vi "DIMPowerSupply.GetRanges.vi"(0 "i ref in":refnum<vi>, 5 "error in (no error)":errorcluster) -> (14 "i ref out":refnum<vi>, 15 "ControlRanges":T1={"deviceMin"=0.0, "deviceMax"=0.0, "numberMin"=0, "numberMax"=0, "U16?"=FALSE, "factor"=1.0} {"deviceMax" format="%.2f"; "deviceMin" format="%.2f"}, 16 "MonitorRanges":T1={"deviceMin"=0.0, "deviceMax"=0.0, "numberMin"=0, "numberMax"=0, "U16?"=FALSE, "factor"=1.0} {"deviceMax" format="%.2f"; "deviceMin" format="%.2f"}, 19 "error out":errorcluster)   [LabVIEW 2014, in "DIMPowerSupply.lvlib"]
doc: "Obtains the ranges of\n1)DeviceMin (minimum voltage value of the power supply output)\n2)DeviceMax (maximum voltage value of the power supply output)\n3)NumberMin (minimum u16 value of the DAC/ADC module)\n4)NumberMax(maximum u16 value of the DAC/ADC module)\n5)ModuleMin (minimum voltage value of the DAC/ADC module)\n6)ModuleMax (maximum voltage value of the DAC/ADC module)"
uses:
  DIMPowerSupply.lvlib
  DIMPowerSupply.ranges type.ctl
  CSCore/BaseProcess/BaseProcess.lvlib
panel:
  in  "Monitor":T1={"deviceMin"=0.0, "deviceMax"=0.0, "numberMin"=0, "numberMax"=0, "U16?"=FALSE, "factor"=1.0} {"deviceMax" format="%.2f"; "deviceMin" format="%.2f"}
  in  "Control":T1={"deviceMin"=0.0, "deviceMax"=0.0, "numberMin"=0, "numberMax"=0, "U16?"=FALSE, "factor"=1.0} {"deviceMax" format="%.2f"; "deviceMin" format="%.2f"}
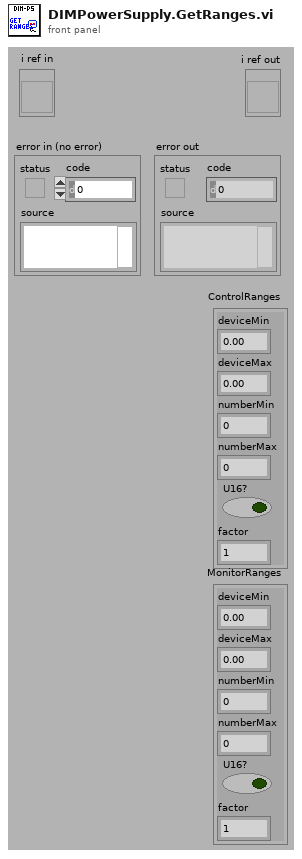
[diagram p1: front panel]
types:
  T1 = typedef "DIMPowerSupply.lvlib/DIMPowerSupply.ranges type.ctl" = cluster{"deviceMin":dbl, "deviceMax":dbl, "numberMin":u16, "numberMax":u16, "U16?":bool, "factor":dbl}
  T2 = typedef "BaseProcess.lvlib/BaseProcess.i attribute.ctl" = cluster{"EventStatus":string, "EventError":i32, "PresetEvtWatchD":i32, "PresetPdcWatchD":i32, "EventTimeout":i32, "PeriodicInterval":i32, "Interface":string[], "Address":string[], "Special":string[], "PeriodicError":i32, "PeriodicStatus":string, "SuperProc":string, "Descriptors":T3[], "CaseRef":refnum<vi>, "PdcRef":refnum<vi>, "Thread Ref":refnum<vi>, "eventErrorID":i32, "eventStatusID":i32, "periodicErrorID":i32, "periodicStatusID":i32, "pdcCtrID":i32}
  T3 = typedef "BaseProcess.lvlib/BaseProcess.descriptor definition.ctl" = cluster{"selector":string, "descriptor":T4}
  T4 = typedef "BaseProcess.lvlib/BaseProcess.descriptor string definition.ctl" = string
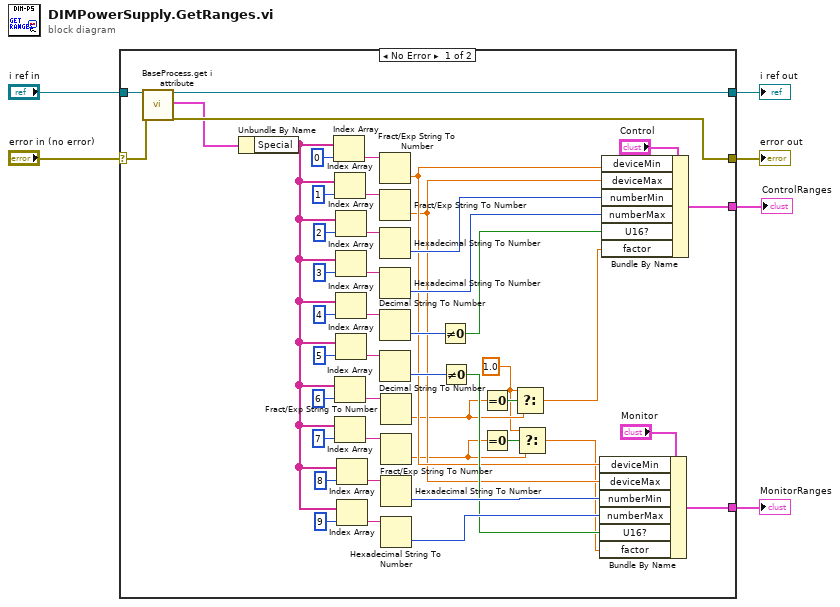
[diagram p0: block diagram]
diagram:
  n1 = case shown="No Error" "error in (no error)" {
    selector: "error in (no error)" -> [w26 w54]
    tunnel: "i ref in" -> [w53 w55]
    tunnel: [w52 w55] -> w5
    tunnel: [w51 w54] -> w4
    tunnel: [w40 _] -> w3
    tunnel: [w29 _] -> w2
    frame No Error {
      w7 = 1.0 ("t")
      n2 = call "BaseProcess.get i attribute.vi"("i ref in"=w53, "error in (no error)"=w26) -> ("i ref out"=w52:refnum<vi>, "i attribute"=w50:T2, "error out"=w51:errorcluster)  [unwired: 15 in]
      n3 = Unbundle By Name(w50) -> ("Special"=w14:string[])
      n4 = Index Array(array=w14, index=0) -> (element=w45:string)
      n5 = Index Array(array=w14, index=1) -> (element=w44:string)
      n6 = Index Array(array=w14, index=6) -> (element=w18:string)
      n7 = Index Array(array=w14, index=7) -> (element=w16:string)
      n8 = Index Array(array=w14, index=2) -> (element=w43:string)
      n9 = Index Array(array=w14, index=3) -> (element=w42:string)
      n10 = Index Array(array=w14, index=4) -> (element=w38:string)
      n11 = Index Array(array=w14, index=5) -> (element=w36:string)
      n12 = Index Array(array=w14, index=8) -> (element=w34:string)
      n13 = Index Array(array=w14, index=9) -> (element=w32:string)
      n14 = Fract/Exp String To Number(string=w45) -> (number=w20:dbl)  [unwired: 3 in, 1 out]
      n15 = Fract/Exp String To Number(string=w44) -> (number=w19:dbl)  [unwired: 3 in, 1 out]
      n16 = Hexadecimal String To Number(string=w43) -> (number=w22:u32)  [unwired: 2 in, 1 out]
      n17 = Hexadecimal String To Number(string=w42) -> (number=w21:u32)  [unwired: 2 in, 1 out]
      n18 = Decimal String To Number(string=w38) -> (number=w31:i32)  [unwired: 2 in, 1 out]
      n19 = Decimal String To Number(string=w36) -> (number=w24:i32)  [unwired: 2 in, 1 out]
      n20 = Fract/Exp String To Number(string=w18) -> (number=w12:dbl)  [unwired: 3 in, 1 out]
      n21 = Fract/Exp String To Number(string=w16) -> (number=w9:dbl)  [unwired: 3 in, 1 out]
      n22 = Hexadecimal String To Number(string=w34) -> (number=w28:u32)  [unwired: 2 in, 1 out]
      n23 = Hexadecimal String To Number(string=w32) -> (number=w27:u32)  [unwired: 2 in, 1 out]
      n24 = Not Equal To 0?(x=w31) -> (x != 0?=w25:bool)
      n25 = Not Equal To 0?(x=w24) -> (x != 0?=w23:bool)
      n26 = Equal To 0?(x=w12) -> (x = 0?=w13:bool)
      n27 = Equal To 0?(x=w9) -> (x = 0?=w10:bool)
      n28 = Select(t=w7, s=w13, f=w12) -> (s? t:f=w11:dbl)
      n29 = Select(t=w7, s=w10, f=w9) -> (s? t:f=w8:dbl)
      n30 = Bundle By Name(cluster="Monitor", "deviceMin"=w20, "deviceMax"=w19, "numberMin"=w28, "numberMax"=w27, "U16?"=w23, "factor"=w8) -> (w29:T1)
      n31 = Bundle By Name(cluster="Control", "deviceMin"=w20, "deviceMax"=w19, "numberMin"=w22, "numberMax"=w21, "U16?"=w25, "factor"=w11) -> (w40:T1)
    }
    frame Error {
    }
  }
  "error out" <- w4
  "i ref out" <- w5
  "ControlRanges" <- w3
  "MonitorRanges" <- w2
